vi "Get Server DLL Path.vi"() -> (0 "Server dll path":path)   [LabVIEW 2019, in "HVC8.lvlib" / "gprc-lvsupport.lvlib"]
uses:
  gprc-lvsupport.lvlib
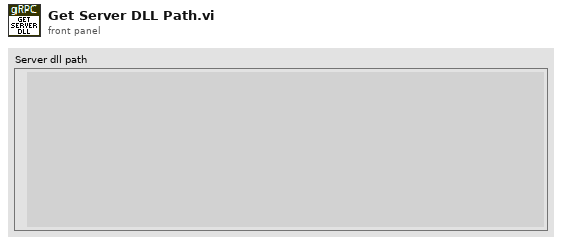
[diagram p1: front panel]
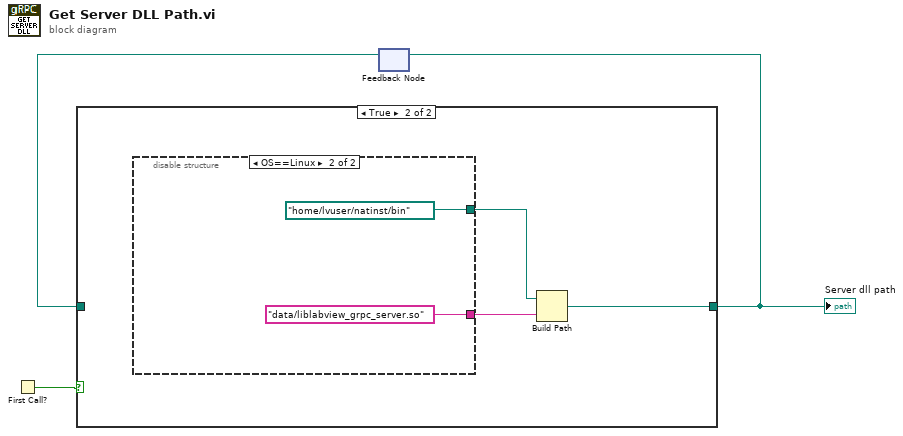
[diagram p0: block diagram]
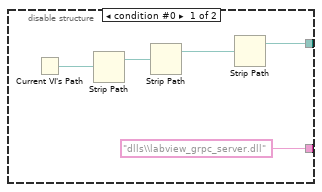
[diagram p3: hidden frame]
diagram:
  n1 = First Call?() -> (First Call?: T/F=w3:bool)
  n2 = feedback #1() -> (w2:path)  [unwired: 1 in]
  n3 = case shown="True" w3 {
    tunnel: [w4 w6] -> w1
    tunnel: w2 -> [w4 _]
    frame False {
    }
    frame True {
      n4 = disable-structure shown="OS==Linux" {
        disable-tunnel: ["dlls\\labview_grpc_server.dll" ("name or relative path") "data/liblabview_grpc_server.so" ("name or relative path")] -> w7
        disable-tunnel: [w8 path "/home/lvuser/natinst/bin" ("stripped path")] -> w5
        frame condition #0 {
          n5 = Current VI's Path() -> (path=w10:path)
          n6 = Strip Path(path=w10) -> (stripped path=w9:path)  [unwired: 1 out]
          n7 = Strip Path(path=w9) -> (stripped path=w11:path)  [unwired: 1 out]
          n8 = Strip Path(path=w11) -> (stripped path=w8:path)  [unwired: 1 out]
        }
        frame condition #1 (active) {
        }
      }
      n9 = Build Path(base path=w5, name or relative path=w7) -> (appended path=w6:path)
    }
  }
  "Server dll path" <- w1
  n10 = feedback-in #1(w1) -> ()
